vi "Wait.vi"(7 "milliseconds to wait":u32=150, 11 "error in (no error)":errorcluster) -> (15 "error out":errorcluster)   [LabVIEW 2014, in "FH 55.lvlib"]
doc: "Wartefunktion, dieses VI wartet bis die angegebene Zeit abgelaufen ist."
uses:
  FH 55.lvlib
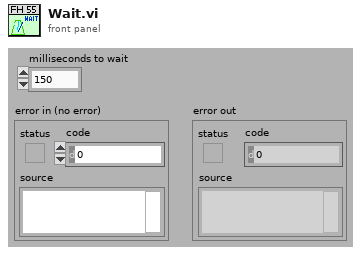
[diagram p1: front panel]
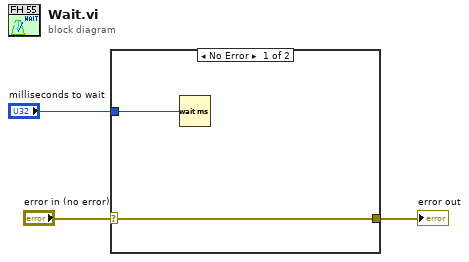
[diagram p0: block diagram]
diagram:
  n1 = case shown="No Error" "error in (no error)" {
    selector: "error in (no error)" -> [w5 w6]
    tunnel: [w5 w6] -> w2
    tunnel: "milliseconds to wait" -> [w4 _]
    frame No Error {
      n2 = Wait (ms)(milliseconds to wait=w4) -> ()  [unwired: 1 out]
    }
    frame Error {
    }
  }
  "error out" <- w2
